vi "Compare Folder Shot Files.vi"(8 "error in (no error)":errorcluster, 10 "Folder Shot File 2":path, 11 "Folder Shot File 1":path) -> (0 "error out":errorcluster)   [LabVIEW 2014, in "SLL File IO.lvlib"]
doc: "Compare two FolderShot Files."
uses:
  SLL File IO.lvlib
panel:
  out "Files Deleted":path[](array[path])
  out "Files Added":path[](array[path])
  out "Files Modified":path[](array[path])
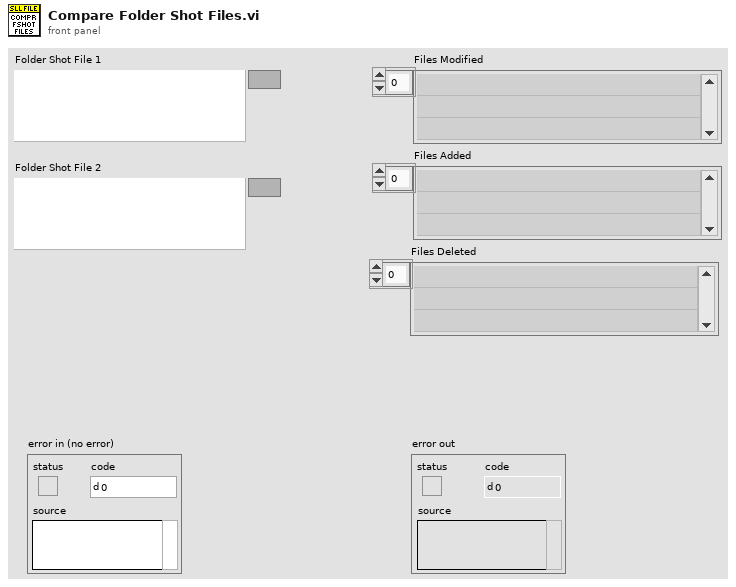
[diagram p1: front panel]
types:
  T1 = typedef "SLL File IO.lvlib/Folder Shot Element.ctl" = cluster{"Abs.Path":path, "Relative Path":path, "MD5":string}
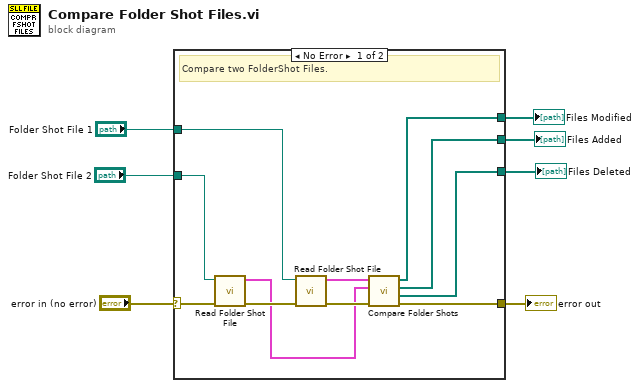
[diagram p0: block diagram]
diagram:
  n1 = case shown="No Error" "error in (no error)" {
    selector: "error in (no error)" -> [w18 w19]
    tunnel: [w13 w19] -> w6
    tunnel: "Folder Shot File 2" -> [w16 _]
    tunnel: "Folder Shot File 1" -> [w14 _]
    tunnel: [w10 _] -> w3
    tunnel: [w9 _] -> w2
    tunnel: [w8 _] -> w1
    frame No Error {
      # "Compare two FolderShot Files."
      n2 = call "Read Folder Shot File.vi"("error in (no error)"=w18, "Log Path"=w16) -> ("error out"=w17:errorcluster, "Folder Shot"=w11:T1[])  [unwired: 8 in]
      n3 = call "Read Folder Shot File.vi"("error in (no error)"=w17, "Log Path"=w14) -> ("error out"=w15:errorcluster, "Folder Shot"=w12:T1[])  [unwired: 8 in]
      n4 = call "Compare Folder Shots.vi"("error in (no error)"=w15, "Folder Shot 2"=w11, "Folder Shot 1"=w12) -> ("error out"=w13:errorcluster, "Files Deleted"=w8:path[], "Files Added"=w9:path[], "Files Modified"=w10:path[])  [unwired: 5 in]
    }
    frame Error {
    }
  }
  "error out" <- w6
  "Files Modified" <- w3
  "Files Added" <- w2
  "Files Deleted" <- w1
